vi "Subtract Float SCTL 40 MHz Latency 0 Pipeline 1.vi"(2 "enable":bool, 3 "y":sgl, 4 "x":sgl) -> (0 "data valid":bool, 1 "x-y":sgl)   [LabVIEW 2014]
uses:
  <vilib>/rvi/IPIntegrationNode/IPINode_Typedef/niFpgaIPINodeSupportedFamilies.ctl
  <vilib>/rvi/IPIntegrationNode/IPINode_Utilities/niFpgaIPINodeSimCore.vi
  <vilib>/rvi/XilinxIP/XIPIN_XNode/niFpgaXIPIN.xnode
  Coregen Zynq/Subtract SCTL L0/xsim.dir/Subtract_SCTL_L0_FF5539BE3A844865B6741F57DA4DC489/xsimk_FF5539BE3A844865B6741F57DA4DC489.dll
  <vilib>/rvi/IPIntegrationNode/IPINode_Xnode/niFpgaIPINode.xnode
  Coregen SPARTAN6/Subtract SCTL L0/Subtract_SCTL_L0_C3ADE5BE76064AA39E7EE6565DE88692.dll
  Coregen KINTEX7/Subtract SCTL L0/xsim.dir/Subtract_SCTL_L0_614AA3EEFEF54D979388EDD38958139F/xsimk_614AA3EEFEF54D979388EDD38958139F.dll
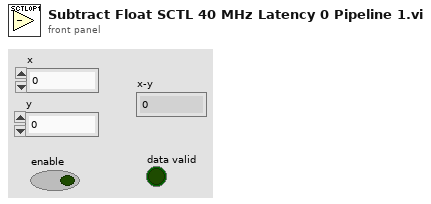
[diagram p1: front panel]
types:
  T1 = typedef "niFpgaIPINodeSupportedFamilies.ctl" = cluster{"unlimited?":bool, "supported targets":string[]}
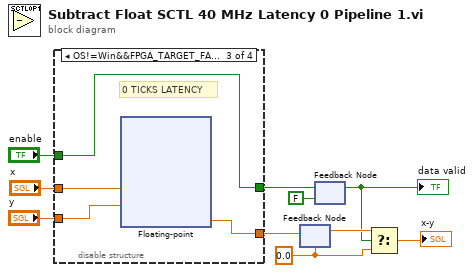
[diagram p0: block diagram]
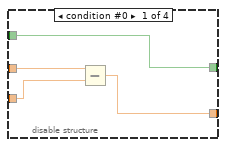
[diagram p2: hidden frame]
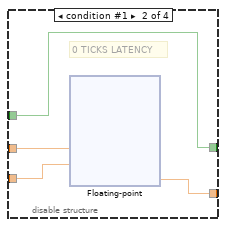
[diagram p3: hidden frame]
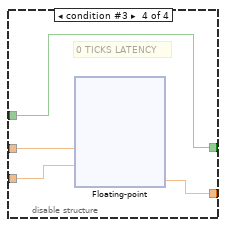
[diagram p4: hidden frame]
diagram:
  w8 = sgl 0.0 ("t")
  n1 = disable-structure shown="OS!=Win&&FPGA_TARGET_FAMILY==ZYNQ" {
    disable-tunnel: "x" -> [w14 w17 w75 w139]
    disable-tunnel: "enable" -> [w12 w18 w76 w140]
    disable-tunnel: [w11 w15 w73 w137] -> w7
    disable-tunnel: [w12 w18 w76 w140] -> w6
    disable-tunnel: "y" -> [w13 w16 w74 w138]
    frame condition #0 {
      n2 = Subtract(x=w14, y=w13) -> (x-y=w11:sgl)
    }
    frame condition #1 {
      # "0 TICKS LATENCY"
      n3 = xnode ("Floating-point")("a"=w17, "b"=w16) -> ("result"=w15:sgl)
    }
    frame condition #2 (active) {
      # "0 TICKS LATENCY"
      n4 = xnode ("Floating-point")("s_axis_a_tdata"=w75, "s_axis_b_tdata"=w74) -> ("m_axis_result_tdata"=w73:sgl)  [unwired: 2 in, 1 out]
    }
    frame condition #3 {
      # "0 TICKS LATENCY"
      n5 = xnode ("Floating-point")("s_axis_a_tdata"=w139, "s_axis_b_tdata"=w138) -> ("m_axis_result_tdata"=w137:sgl)  [unwired: 2 in, 1 out]
    }
  }
  n6 = feedback #1(w8) -> (w10:sgl)
  n7 = feedback-in #1(w7) -> ()
  n8 = feedback #2(FALSE ("reset")) -> (w2:bool)
  "data valid" <- w2
  n9 = feedback-in #2(w6) -> ()
  n10 = Select(t=w10, s=w2, f=w8) -> (s? t:f=→"x-y":sgl)
